vi "AE - Bluetooth Pair All.vi"(8 "error in (no error)":errorcluster) -> (0 "error out":errorcluster, 3 "Number of wiimotes paired":i32)   [LabVIEW 2010]
uses:
  AE Cores/AE - Bluetooth Enum.ctl
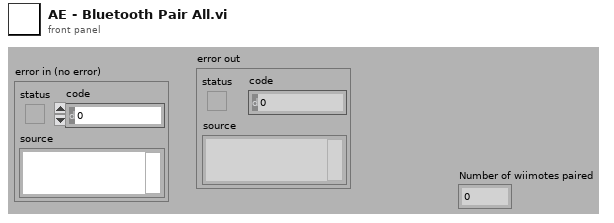
[diagram p1: front panel]
types:
  T1 = typedef "AE - Bluetooth Enum.ctl" = enum16{"Initialise", "Pair All Wiimotes", "Connect All Wiimotes", "Set Rumble", "Set LED", "Get Button + Acc Data", "Get IR Data", "Get Battery", "Get Wiimote Reference", "Reorder Wiimotes", "devReport"}
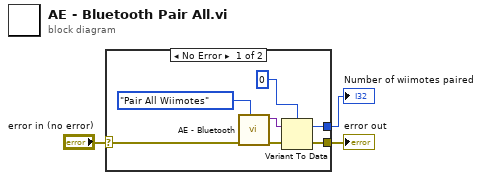
[diagram p0: block diagram]
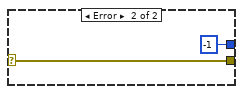
[diagram p2: hidden frame]
diagram:
  n1 = case shown="No Error" "error in (no error)" {
    selector: "error in (no error)" -> [w9 w12]
    tunnel: [w4 w12] -> w2
    tunnel: [w7 -1] -> w1
    frame No Error {
      n2 = call "AE - Bluetooth.vi"("Enum"=AE_-_Bluetooth_Enum."Pair All Wiimotes", "error in (no error)"=w9) -> ("error out"=w8:errorcluster, "Variant Out"=w5:variant)  [unwired: 7 in, 1 out]
      n3 = Variant To Data(error in=w8, Variant=w5, type=0) -> (error out=w4:errorcluster, data=w7:i32)
    }
    frame Error {
    }
  }
  "error out" <- w2
  "Number of wiimotes paired" <- w1
